vi "Set LED and Filter Settings.vi"(8 "error in (no error)":errorcluster, 9 "Filter Values":T1(array[cluster]), 10 "Laser Values":T2(array[cluster]), 11 "Settings in":refnum<class "Settings.lvclass">) -> (0 "error out":errorcluster, 3 "Settings out":refnum<class "Settings.lvclass">)   [LabVIEW 2010, in "Settings.lvclass"]
uses:
  Settings.lvclass
  Settings.lvclass/Settings.ctl
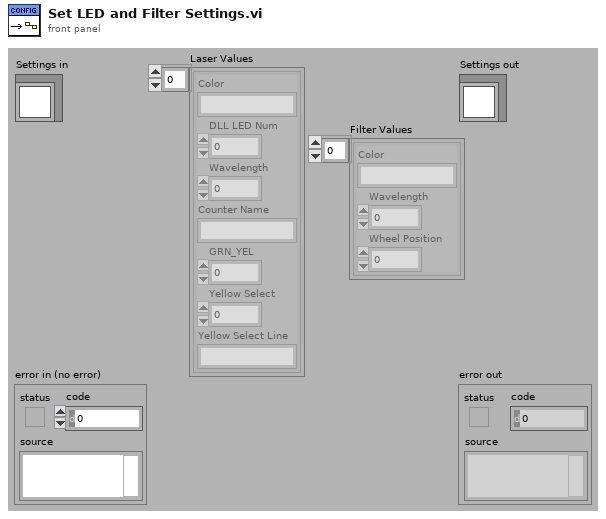
[diagram p1: front panel]
types:
  T1 = cluster{"Color":string, "Wavelength":i32, "Wheel Position":i32}[]
  T2 = cluster{"Color":string, "DLL LED Num":i32, "Wavelength":i32, "Counter Name":string, "GRN_YEL":i32, "Yellow Select":i32, "Yellow Select Line":string}[]
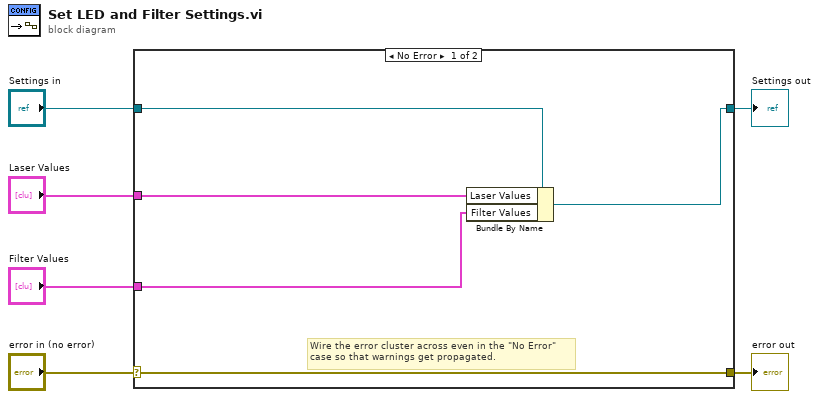
[diagram p0: block diagram]
diagram:
  n1 = case shown="No Error" "error in (no error)" {
    selector: "error in (no error)" -> [w11 w13]
    tunnel: [w11 w13] -> w5
    tunnel: [w9 w12] -> w3
    tunnel: "Settings in" -> [w10 w12]
    tunnel: "Laser Values" -> [w8 _]
    tunnel: "Filter Values" -> [w7 _]
    frame No Error {
      # "Wire the error cluster across even in the \"No Error\"\ncase so that warnings get propagated."
      n2 = Bundle By Name(cluster=w10, "Laser Values"=w8, "Filter Values"=w7) -> (w9:refnum<class "Settings.lvclass">)
    }
    frame Error {
    }
  }
  "error out" <- w5
  "Settings out" <- w3
